vi "Convert Line to Obj Data.vi"(5 "error in (no error)":errorcluster, 7 "Channel Lines info":T2(array[cluster]), 9 "Line text":string[](array[string])) -> (13 "FRF":T1(array[cluster]), 19 "error out":errorcluster)   [LabVIEW 2020, in "Nastran PCH.lvclass"]
uses:
  Nastran PCH.lvclass
  protected/ObjectAttributes.ctl
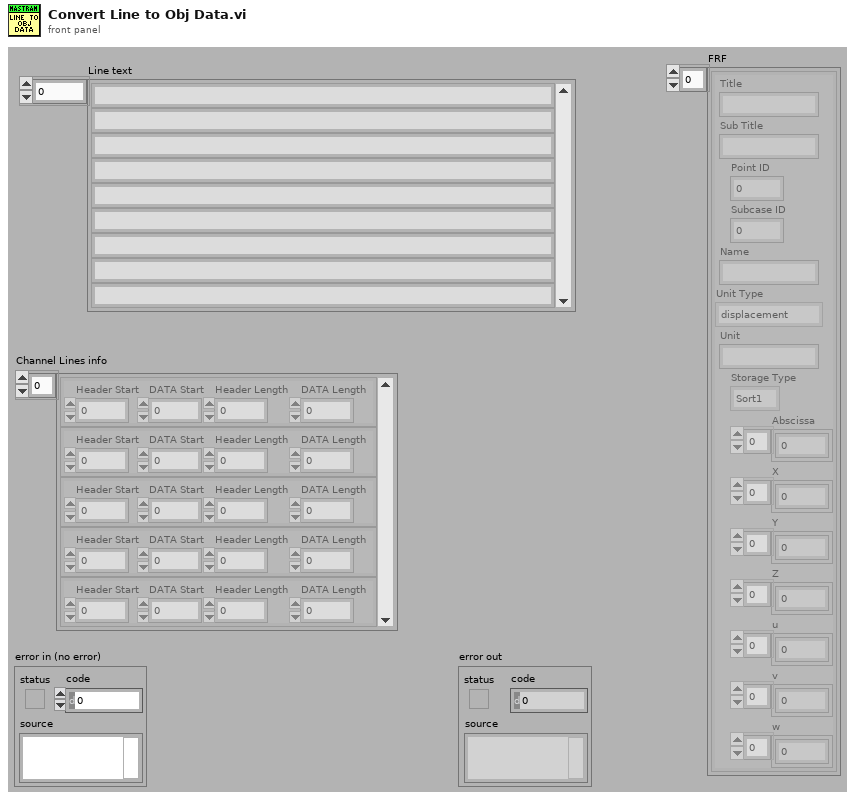
[diagram p1: front panel]
types:
  T1 = cluster{"Title":string, "Sub Title":string, "Point ID":i32, "Subcase ID":i32, "Name":string, "Unit Type":enum16{"displacement", "velocity", "acceleration"}, "Unit":string, "Storage Type":enum16{"Sort1", "Sort2"}, "Abscissa":dbl[], "X":cdb[], "Y":cdb[], "Z":cdb[], "u":cdb[], "v":cdb[], "w":cdb[]}[]
  T2 = cluster{"Header Start":i32, "DATA Start":i32, "Header Length":i32, "DATA Length":i32}[]
  T3 = typedef "Nastran PCH.lvclass/ObjectAttributes.ctl" = cluster{"FRF":cluster{"Title":string, "Sub Title":string, "Point ID":i32, "Subcase ID":i32, "Name":string, "Unit Type":enum16{"displacement", "velocity", "acceleration"}, "Unit":string, "Storage Type":enum16{"Sort1", "Sort2"}, "Abscissa":dbl[], "X":cdb[], "Y":cdb[], "Z":cdb[], "u":cdb[], "v":cdb[], "w":cdb[]}[]}
  T4 = enum16{"displacement", "velocity", "acceleration"}
  T5 = cluster{"Title":string, "Sub Title":string, "Point ID":i32, "Subcase ID":i32, "Name":string, "Unit Type":enum16{"displacement", "velocity", "acceleration"}, "Unit":string, "Storage Type":enum16{"Sort1", "Sort2"}, "Abscissa":dbl[], "X":cdb[], "Y":cdb[], "Z":cdb[], "u":cdb[], "v":cdb[], "w":cdb[]}
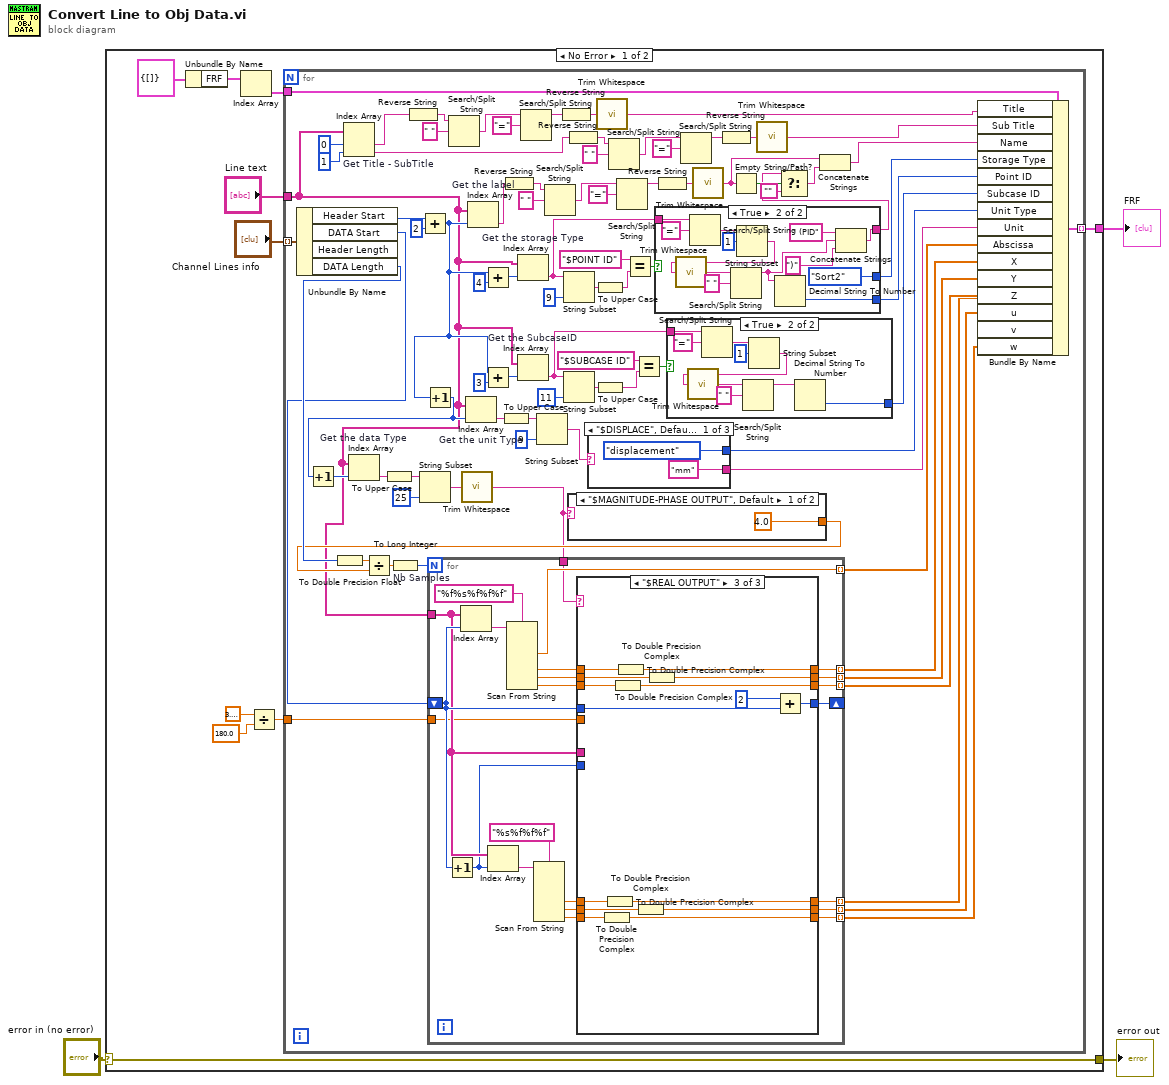
[diagram p0: block diagram]
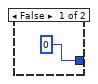
[diagram p2: hidden frame]
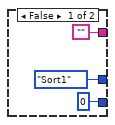
[diagram p3: hidden frame]
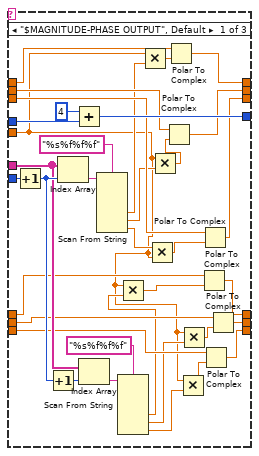
[diagram p4: hidden frame]
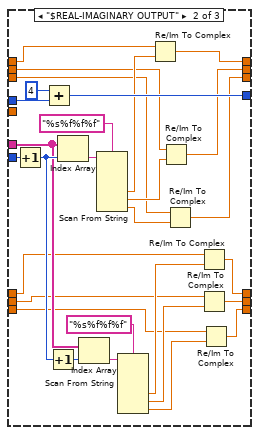
[diagram p5: hidden frame]
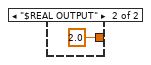
[diagram p6: hidden frame]
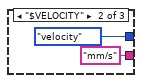
[diagram p7: hidden frame]
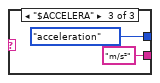
[diagram p8: hidden frame]
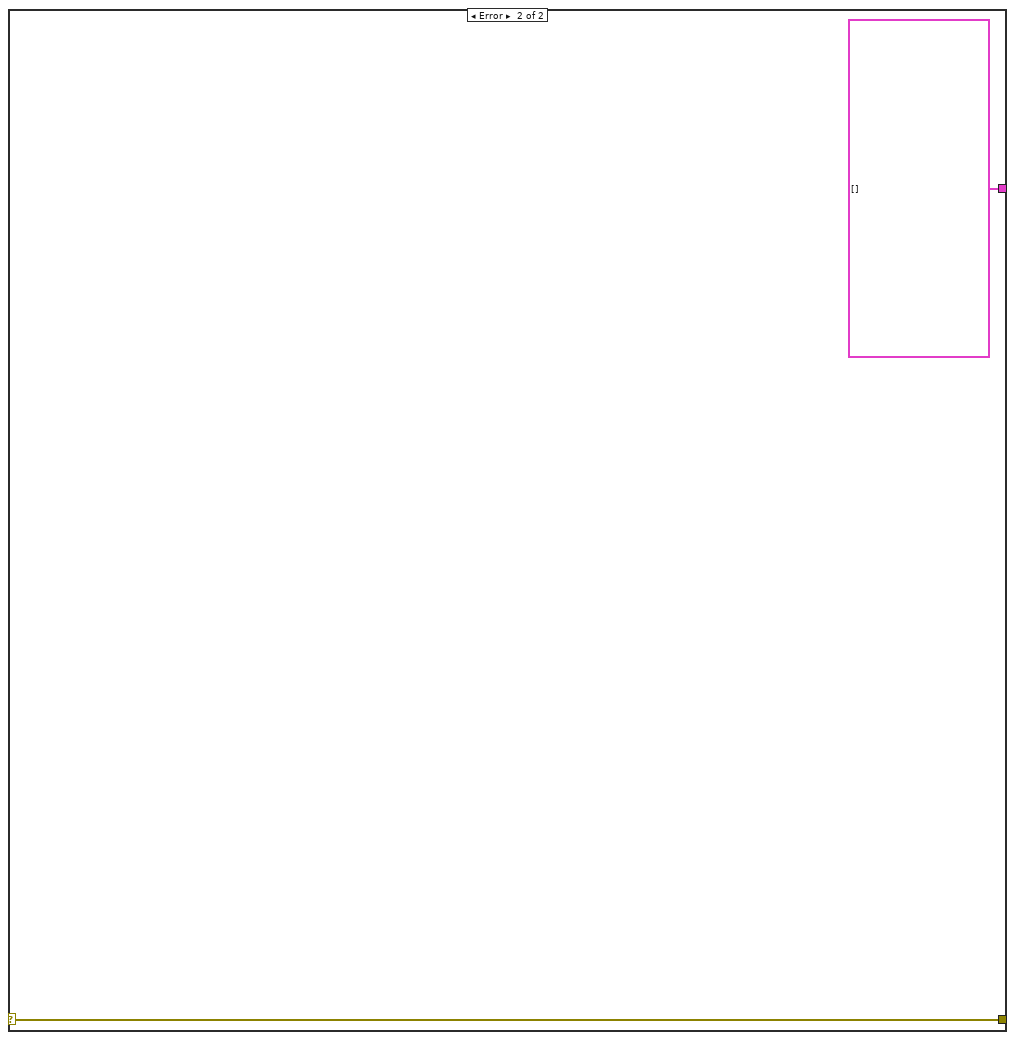
[diagram p9: hidden frame]
diagram:
  n1 = case shown="No Error" "error in (no error)" {
    selector: "error in (no error)" -> [w13 w236]
    tunnel: [w13 w236] -> w2
    tunnel: [w4 T1 []] -> w1
    frame No Error {
      n2 = Unbundle By Name(T3 {"FRF"=[]} ("Base class")) -> ("FRF"=w5:T1)
      n3 = Index Array(array=w5) -> (element=w8:T5)  [unwired: 1 in]
      n4 = Divide(x=3.141592653589793, y=180.0) -> (x/y=w12:dbl)
      n5 = for {
        tunnel: "Channel Lines info" -> [w97] mode=indexing
        tunnel: "Line text" -> [w18]
        tunnel: w8 -> [w92]
        tunnel: [w67] -> w4 mode=indexing
        tunnel: w12 -> [w66]
        n6 = Unbundle By Name(w97) -> ("Header Start"=w96:i32, "DATA Start"=w76:i32, "DATA Length"=w81:i32)  [unwired: 1 out]
        n7 = To Double Precision Float(number=w81) -> (double precision float=w78:dbl)
        n8 = Index Array "Get Title - SubTitle"(array=w18, index #1=0 ("index"), index #2=1 ("index")) -> (element #1=w36:string, element #2=w35:string)
        n9 = Reverse String(1:w36) -> (0:w45:string)
        n10 = Add(x=w96, y=2) -> (x+y=w19:i32)
        n11 = Increment(x=w19) -> (x+1=w86:i32)
        n12 = Increment(x=w86) -> (x+1=w87:i32)
        n13 = Index Array "Get the data Type"(array=w18, index=w87) -> (element=w83:string)
        n14 = To Upper Case(1:w83) -> (0:w84:string)
        n15 = String Subset(string=w84, length (rest)=25 ("length (rest)")) -> (substring=w82:string)  [unwired: 1 out]
        n16 = Search/Split String(string=w45, search string/char (-)=" ") -> (match + rest of string=w46:string)  [unwired: 3 out]
        n17 = call <vilib>:"Trim Whitespace.vi"("string"=w82) -> ("trimmed string"=w74:string)  [unwired: 1 in]
        n18 = Index Array "Get the unit Type"(array=w18, index=w86) -> (element=w91:string)
        n19 = Index Array "Get the label"(array=w18, index=w19) -> (element=w94:string)
        n20 = Add(x=w19, y=4) -> (x+y=w58:i32)
        n21 = Add(x=w19, y=3) -> (x+y=w21:i32)
        n22 = To Upper Case(1:w91) -> (0:w90:string)
        n23 = Reverse String(1:w94) -> (0:w64:string)
        n24 = Index Array "Get the storage Type"(array=w18, index=w58) -> (element=w52:string)
        n25 = Index Array "Get the SubcaseID"(array=w18, index=w21) -> (element=w15:string)
        n26 = Search/Split String(string=w46, search string/char (-)="=") -> (substring before match=w48:string)  [unwired: 3 out]
        n27 = String Subset(string=w90, length (rest)=9 ("length (rest)")) -> (substring=w88:string)  [unwired: 1 out]
        n28 = Search/Split String(string=w64, search string/char (-)=" ") -> (match + rest of string=w63:string)  [unwired: 3 out]
        n29 = Reverse String(1:w48) -> (0:w47:string)
        n30 = String Subset(string=w52, length (rest)=9 ("length (rest)")) -> (substring=w55:string)  [unwired: 1 out]
        n31 = String Subset(string=w15, length (rest)=11 ("length (rest)")) -> (substring=w23:string)  [unwired: 1 out]
        n32 = Reverse String(1:w35) -> (0:w40:string)
        n33 = case shown="\"$MAGNITUDE-PHASE OUTPUT\", Default" w74 {
          tunnel: [4.0 2.0] -> w79
          frame "$MAGNITUDE-PHASE OUTPUT", Default {
          }
          frame "$REAL OUTPUT" {
          }
        }
        n34 = Divide(x=w78, y=w79) -> (x/y=w80:dbl)
        n35 = To Long Integer "Nb Samples"(number=w80) -> (32bit integer=w77:i32)
        n36 = for {
          N: w77 -> [_]
          shift-right: [w142] -> _
          shift-left: w76 -> [w139]
          tunnel: w18 -> [w126]
          tunnel: [w144] -> w75 mode=indexing
          tunnel: w74 -> [w143]
          tunnel: [w137] -> w73 mode=indexing
          tunnel: [w135] -> w72 mode=indexing
          tunnel: [w133] -> w71 mode=indexing
          tunnel: [w129] -> w70 mode=indexing
          tunnel: [w128] -> w69 mode=indexing
          tunnel: [w127] -> w68 mode=indexing
          tunnel: w66 -> [w124]
          n37 = Increment(x=w139) -> (x+1=w125:i32)
          n38 = Index Array(array=w126, index=w139) -> (element=w145:string)
          n39 = Index Array(array=w126, index=w125) -> (element=w141:string)
          n40 = Scan From String(format string="%f%s%f%f%f", input string=w145) -> (output 1=w144:dbl, output 3=w138:dbl, output 4=w136:dbl, output 5=w134:dbl)  [unwired: 2 in, 9 out]
          n41 = Scan From String(format string="%s%f%f%f", input string=w141) -> (output 2=w132:dbl, output 3=w131:dbl, output 4=w130:dbl)  [unwired: 2 in, 8 out]
          n42 = case shown="\"$REAL OUTPUT\"" w143 {
            tunnel: [w181 w210 w226] -> w142
            tunnel: w139 -> [w180 w209 w224]
            tunnel: w138 -> [w171 w200 w223]
            tunnel: [w170 w198 w222] -> w137
            tunnel: w136 -> [w169 w197 w220]
            tunnel: [w168 w195 w221] -> w135
            tunnel: w134 -> [w167 w194 w219]
            tunnel: [w166 w192 w218] -> w133
            tunnel: w132 -> [w164 w190 w217]
            tunnel: w131 -> [w162 w187 w216]
            tunnel: w130 -> [w160 w184 w215]
            tunnel: [w165 w191 w214] -> w129
            tunnel: [w163 w188 w213] -> w128
            tunnel: [w161 w185 w212] -> w127
            tunnel: w126 -> [w172 w201 _]
            tunnel: w125 -> [w177 w206 _]
            tunnel: w124 -> [w148 _ _]
            frame "$MAGNITUDE-PHASE OUTPUT", Default {
              n43 = Increment(x=w177) -> (x+1=w173:i32)
              n44 = Increment(x=w173) -> (x+1=w176:i32)
              n45 = Index Array(array=w172, index=w173) -> (element=w178:string)
              n46 = Add(x=4, y=w180) -> (x+y=w181:i32)
              n47 = Index Array(array=w172, index=w176) -> (element=w175:string)
              n48 = Scan From String(format string="%s%f%f%f", input string=w178) -> (output 2=w158:dbl, output 3=w157:dbl, output 4=w154:dbl)  [unwired: 2 in, 8 out]
              n49 = Scan From String(format string="%s%f%f%f", input string=w175) -> (output 2=w153:dbl, output 3=w151:dbl, output 4=w149:dbl)  [unwired: 2 in, 8 out]
              n50 = Multiply(x=w148, y=w153) -> (x*y=w152:dbl)
              n51 = Multiply(x=w148, y=w158) -> (x*y=w159:dbl)
              n52 = Multiply(x=w154, y=w148) -> (x*y=w155:dbl)
              n53 = Multiply(x=w148, y=w157) -> (x*y=w156:dbl)
              n54 = Polar To Complex(1:w156, 2:w169) -> (0:w168:cdb)
              n55 = Polar To Complex(1:w159, 2:w171) -> (0:w170:cdb)
              n56 = Multiply(x=w148, y=w149) -> (x*y=w147:dbl)
              n57 = Multiply(x=w148, y=w151) -> (x*y=w150:dbl)
              n58 = Polar To Complex(1:w152, 2:w164) -> (0:w165:cdb)
              n59 = Polar To Complex(1:w155, 2:w167) -> (0:w166:cdb)
              n60 = Polar To Complex(1:w147, 2:w160) -> (0:w161:cdb)
              n61 = Polar To Complex(1:w150, 2:w162) -> (0:w163:cdb)
            }
            frame "$REAL-IMAGINARY OUTPUT" {
              n62 = Increment(x=w206) -> (x+1=w202:i32)
              n63 = Add(x=4, y=w209) -> (x+y=w210:i32)
              n64 = Increment(x=w202) -> (x+1=w205:i32)
              n65 = Index Array(array=w201, index=w202) -> (element=w207:string)
              n66 = Index Array(array=w201, index=w205) -> (element=w204:string)
              n67 = Scan From String(format string="%s%f%f%f", input string=w207) -> (output 2=w199:dbl, output 3=w196:dbl, output 4=w193:dbl)  [unwired: 2 in, 8 out]
              n68 = Scan From String(format string="%s%f%f%f", input string=w204) -> (output 2=w189:dbl, output 3=w186:dbl, output 4=w183:dbl)  [unwired: 2 in, 8 out]
              n69 = Re/Im To Complex(1:w199, 2:w200) -> (0:w198:cdb)
              n70 = Re/Im To Complex(1:w196, 2:w197) -> (0:w195:cdb)
              n71 = Re/Im To Complex(1:w193, 2:w194) -> (0:w192:cdb)
              n72 = Re/Im To Complex(1:w189, 2:w190) -> (0:w191:cdb)
              n73 = Re/Im To Complex(1:w186, 2:w187) -> (0:w188:cdb)
              n74 = Re/Im To Complex(1:w183, 2:w184) -> (0:w185:cdb)
            }
            frame "$REAL OUTPUT" {
              n75 = To Double Precision Complex(1:w215) -> (0:w212:cdb)
              n76 = To Double Precision Complex(1:w217) -> (0:w214:cdb)
              n77 = To Double Precision Complex(1:w219) -> (0:w218:cdb)
              n78 = To Double Precision Complex(1:w223) -> (0:w222:cdb)
              n79 = To Double Precision Complex(1:w216) -> (0:w213:cdb)
              n80 = To Double Precision Complex(1:w220) -> (0:w221:cdb)
              n81 = Add(x=2, y=w224) -> (x+y=w226:i32)
            }
          }
        }
        n82 = case shown="\"$DISPLACE\", Default" w88 {
          tunnel: [T4."displacement" ("Type") T4."velocity" ("Type") T4."acceleration" ("Type")] -> w60
          tunnel: ["mm" ("string") "mm/s" ("string") "m/s²" ("string")] -> w51
          frame "$DISPLACE", Default {
          }
          frame "$VELOCITY" {
          }
          frame "$ACCELERA" {
          }
        }
        n83 = To Upper Case(1:w55) -> (0:w54:string)
        n84 = To Upper Case(1:w23) -> (0:w24:string)
        n85 = call <vilib>:"Trim Whitespace.vi"("string"=w47) -> ("trimmed string"=w34:string)  [unwired: 1 in]
        n86 = Search/Split String(string=w40, search string/char (-)=" ") -> (match + rest of string=w39:string)  [unwired: 3 out]
        n87 = Search/Split String(string=w63, search string/char (-)="=") -> (substring before match=w61:string)  [unwired: 3 out]
        n88 = Equal?(x="$POINT ID", y=w54) -> (x = y?=w53:bool)
        n89 = Equal?(x="$SUBCASE ID", y=w24) -> (x = y?=w16:bool)
        n90 = case shown="True" w53 {
          tunnel: [enum16{"Sort1", "Sort2"}."Sort1" ("Storage Type") enum16{"Sort1", "Sort2"}."Sort2" ("Storage Type")] -> w26
          tunnel: ["" w122] -> w30
          tunnel: w52 -> [_ w119]
          tunnel: [0 w111] -> w25
          frame False {
          }
          frame True {
            n91 = Search/Split String(string=w119, search string/char (-)="=") -> (match + rest of string=w118:string)  [unwired: 3 out]
            n92 = String Subset(string=w118, offset (0)=1) -> (substring=w115:string)  [unwired: 1 out]
            n93 = call <vilib>:"Trim Whitespace.vi"("string"=w115) -> ("trimmed string"=w113:string)  [unwired: 1 in]
            n94 = Search/Split String(string=w113, search string/char (-)=" ") -> (substring before match=w112:string)  [unwired: 3 out]
            n95 = Decimal String To Number(string=w112) -> (number=w111:i32)  [unwired: 3 out]
            n96 = Concatenate Strings(" (PID" ("string"), w112, ")" ("string")) -> (w122:string)
          }
        }
        n97 = Reverse String(1:w61) -> (0:w62:string)
        n98 = case shown="True" w16 {
          tunnel: w15 -> [_ w107]
          tunnel: [0 w99] -> w14
          frame False {
          }
          frame True {
            n99 = Search/Split String(string=w107, search string/char (-)="=") -> (match + rest of string=w106:string)  [unwired: 3 out]
            n100 = String Subset(string=w106, offset (0)=1) -> (substring=w103:string)  [unwired: 1 out]
            n101 = call <vilib>:"Trim Whitespace.vi"("string"=w103) -> ("trimmed string"=w101:string)  [unwired: 1 in]
            n102 = Search/Split String(string=w101, search string/char (-)=" ") -> (substring before match=w100:string)  [unwired: 3 out]
            n103 = Decimal String To Number(string=w100) -> (number=w99:i32)  [unwired: 3 out]
          }
        }
        n104 = Search/Split String(string=w39, search string/char (-)="=") -> (substring before match=w37:string)  [unwired: 3 out]
        n105 = call <vilib>:"Trim Whitespace.vi"("string"=w62) -> ("trimmed string"=w32:string)  [unwired: 1 in]
        n106 = Reverse String(1:w37) -> (0:w38:string)
        n107 = Empty String/Path?(string/path=w32) -> (empty?=w31:bool)
        n108 = call <vilib>:"Trim Whitespace.vi"("string"=w38) -> ("trimmed string"=w33:string)  [unwired: 1 in]
        n109 = Select(t=w30, s=w31, f="") -> (s? t:f=w28:string)
        n110 = Concatenate Strings(w32, w28) -> (w27:string)
        n111 = Bundle By Name(cluster=w92, "Title"=w34, "Sub Title"=w33, "Name"=w27, "Storage Type"=w26, "Point ID"=w25, "Subcase ID"=w14, "Unit Type"=w60, "Unit"=w51, "Abscissa"=w75, "X"=w73, "Y"=w72, "Z"=w71, "u"=w70, "v"=w69, "w"=w68) -> (w67:T5)
      }
    }
    frame Error {
    }
  }
  "error out" <- w2
  "FRF" <- w1
